vi "Open.vi"(8 "error in (no error)":errorcluster, 11 "NI Digital in":refnum<class "NI Analog Out.lvclass">) -> (0 "error out":errorcluster, 3 "NI Digital out":refnum<class "NI Analog Out.lvclass">)   [LabVIEW 2018, in "NI Analog Out.lvclass"]
doc: "NI Analog Out.lvclass:Open.vi\n\nThis is the Open VI for the NI Analog Out class. It configures an analog out device.\n\nInstrument Communication Module Version 1.0\nOctober, 2020 Original Code Consulting Davita Bird\n www.originalcode.com"
uses:
  NI Analog Out.lvclass
  NI Analog Out.lvclass/NI Analog Out.ctl
  <vilib>/DAQmx/create/channels.llb/DAQmx Create Channel (AO-Voltage-Basic).vi
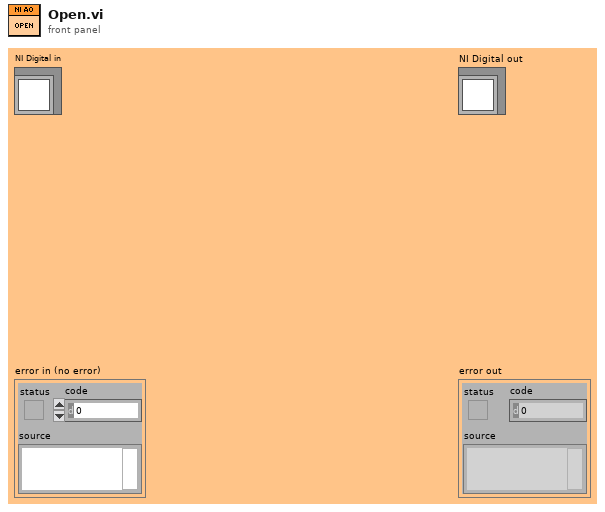
[diagram p1: front panel]
types:
  T1 = typedef "NI Analog Channel Range.ctl" = enum16{"-10.0 to 10.0 V", "-5.0 to 5.0 V", "-2.0 to 2.0 V", "-1.0 to 1.0 V", "-0.5 to 0.5 V", "-0.2 to 0.2 V", "-0.1 to 0.1 V", "0 to 10 V", "0 to 5 V", "0 to 2 V", "0 to 1 V", "0 to 0.5 V", "0 to 0.2 V", "0 to 0.1 V"}
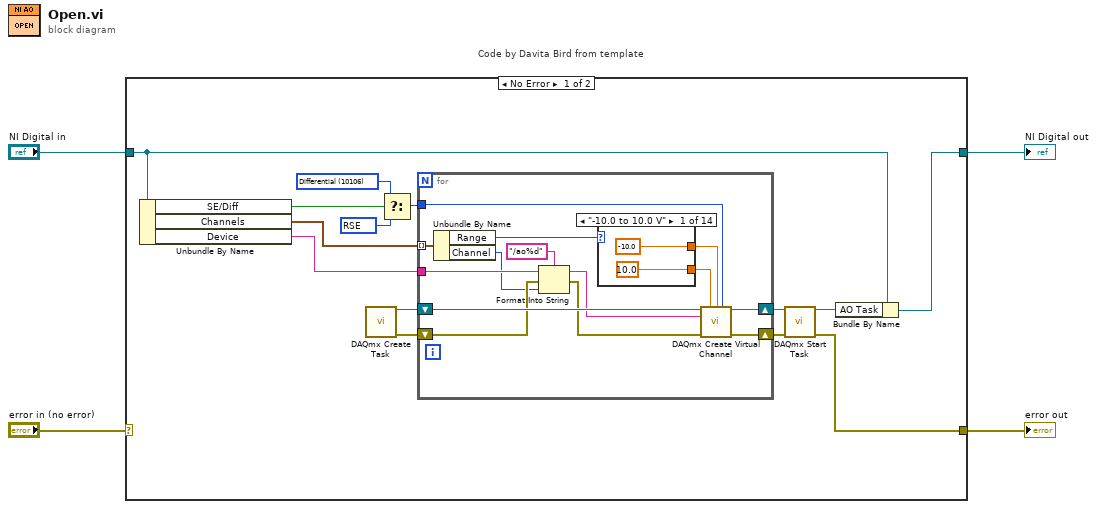
[diagram p0: block diagram]
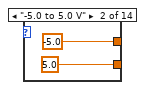
[diagram p2: hidden frame]
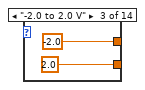
[diagram p3: hidden frame]
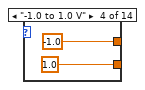
[diagram p4: hidden frame]
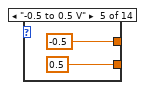
[diagram p5: hidden frame]
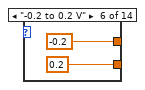
[diagram p6: hidden frame]
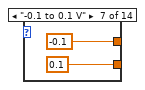
[diagram p7: hidden frame]
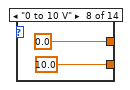
[diagram p8: hidden frame]
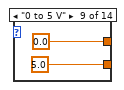
[diagram p9: hidden frame]
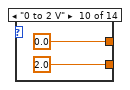
[diagram p10: hidden frame]
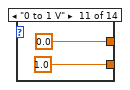
[diagram p11: hidden frame]
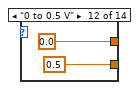
[diagram p12: hidden frame]
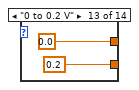
[diagram p13: hidden frame]
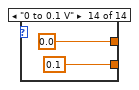
[diagram p14: hidden frame]
diagram:
  n1 = case "Code by Davita Bird from template" shown="No Error" "error in (no error)" {
    selector: "error in (no error)" -> [_ w62]
    tunnel: [w6 w62] -> w3
    tunnel: [w17 w61] -> w2
    tunnel: "NI Digital in" -> [w18 w61]
    frame No Error {
      w15 = 10083 items=["default"=-1, "RSE"=10083, "NRSE"=10078, "Differential"=10106, "Pseudodifferential"=12529] ("input terminal configuration")
      w16 = 10106 items=["default"=-1, "RSE"=10083, "NRSE"=10078, "Differential"=10106, "Pseudodifferential"=12529] ("input terminal configuration")
      n2 = Unbundle By Name(w18) -> ("SE/Diff"=w14:bool, "Channels"=w5:cluster{"Channel":i32, "Range":T1}[], "Device"=w11:string)
      n3 = call <vilib>:"DAQmx Create Task.vi"() -> ("task out"=w13:refnum<k21>, "error out"=w12:errorcluster)  [unwired: 5 in, 9 out]
      n4 = Select(t=w16, s=w14, f=w15) -> (s? t:f=w10:i32)
      n5 = for {
        shift-right: [w23] -> w8
        shift-left: w13 -> [w27]
        shift-right: [w22] -> w9
        shift-left: w12 -> [w26]
        tunnel: w11 -> [w31]
        tunnel: w10 -> [w28]
        tunnel: w5 -> [w21] mode=indexing
        n6 = Unbundle By Name(w21) -> ("Range"=w19:T1, "Channel"=w20:i32)
        n7 = Format Into String(format string="/ao%d", initial string=w31, error in=w26, w20) -> (resulting string=w24:string, error out=w25:errorcluster)
        n8 = case shown="\"-10.0 to 10.0 V\"" w19 {
          tunnel: [10.0 5.0 2.0 1.0 0.5 0.2 0.1 10.0 5.0 2.0 1.0 0.5 0.2 0.1] -> w30
          tunnel: [-10.0 -5.0 -2.0 -1.0 -0.5 -0.2 -0.1 0.0 0.0 0.0 0.0 0.0 0.0 0.0] -> w29
          frame "-10.0 to 10.0 V" {
          }
          frame "-5.0 to 5.0 V" {
          }
          frame "-2.0 to 2.0 V" {
          }
          frame "-1.0 to 1.0 V" {
          }
          frame "-0.5 to 0.5 V" {
          }
          frame "-0.2 to 0.2 V" {
          }
          frame "-0.1 to 0.1 V" {
          }
          frame "0 to 10 V" {
          }
          frame "0 to 5 V" {
          }
          frame "0 to 2 V" {
          }
          frame "0 to 1 V" {
          }
          frame "0 to 0.5 V" {
          }
          frame "0 to 0.2 V" {
          }
          frame "0 to 0.1 V" {
          }
        }
        n9 = call-poly <vilib>:"DAQmx Create Virtual Channel.vi"("task in"=w27, "maximum value"=w30, "minimum value"=w29, "output terminal configuration"=w28, "physical channels"=w24, "error in"=w25) -> ("task out"=w23:refnum<k21>, "error out"=w22:errorcluster)  [unwired: 3 in, 5 out]
      }
      n10 = call <vilib>:"DAQmx Start Task.vi"("task/channels in"=w8, "error in"=w9) -> ("task out"=w7:refnum<k21>, "error out"=w6:errorcluster)  [unwired: 12 in]
      n11 = Bundle By Name(cluster=w18, "AO Task"=w7) -> (w17:refnum<class "NI Analog Out.lvclass">)
    }
    frame Error {
    }
  }
  "error out" <- w3
  "NI Digital out" <- w2
